vi "Write Scan Log.vi"(8 "error in (no error)":errorcluster, 10 "File Name":string, 11 "Model in":refnum<class "Model.lvclass">) -> (0 "error out":errorcluster, 3 "Model out":refnum<class "Model.lvclass">)   [LabVIEW 2015, in "Model.lvclass"]
uses:
  Model.lvclass
  Typedefs/Write Data File Arguments.ctl
  Typedefs/Write Log Message Arguments.ctl
  Model.lvclass/Model.ctl
  Test Log/Test Log/Test Log.lvclass
  Typedefs/FAMT Typedefs.lvlib
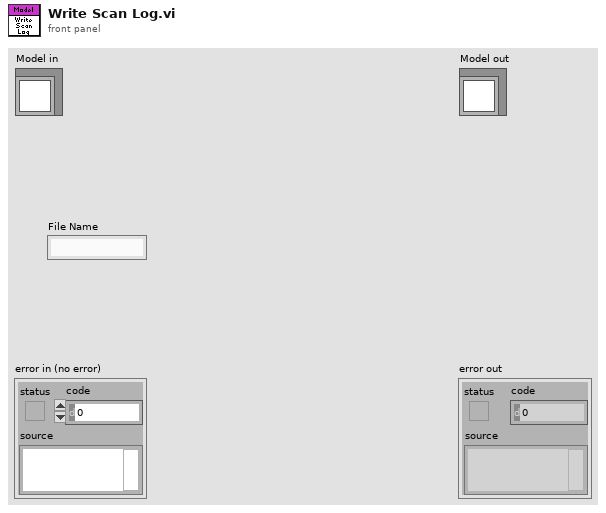
[diagram p1: front panel]
types:
  T1 = typedef "FAMT Typedefs.lvlib/Write Log Message Arguments.ctl" = cluster{"Description":string, "Data File":string}
  T2 = typedef "FAMT Typedefs.lvlib/Write Data File Arguments.ctl" = cluster{"File Name":string, "Output":string[]}
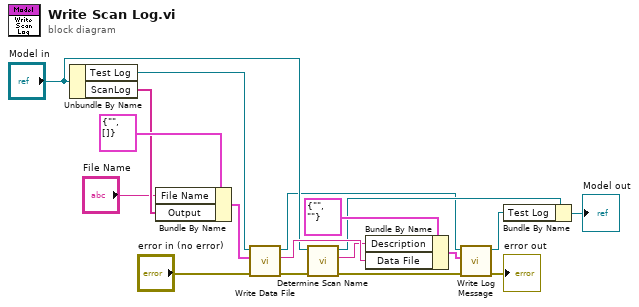
[diagram p0: block diagram]
diagram:
  n1 = Unbundle By Name("Model in") -> ("Test Log"=w18:refnum<class "Test Log.lvclass">, "ScanLog"=w14:string[])
  n2 = Bundle By Name(cluster=T2 {"File Name"="", "Output"=[]} ("WriteDataFileInput"), "File Name"="File Name", "Output"=w14) -> (w15:T2)
  n3 = call-dynamic "Write Data File.vi"("error in (no error)"="error in (no error)", "Write Data File Arguments"=w15, "Test Log in"=w18) -> ("error out"=w3:errorcluster, "Relative Path"=w10:string, "Test Log out"=w6:refnum<class "Test Log.lvclass">)  [unwired: 6 in]
  n4 = call "Determine Scan Name.vi"("error in (no error)"=w3, "Model in"="Model in") -> ("error out"=w2:errorcluster, "Scan Name"=w9:string, "Model out"=w7:refnum<class "Model.lvclass">)  [unwired: 7 in]
  n5 = Bundle By Name(cluster=T1 {"Description"="", "Data File"=""} ("WriteLogMessageInput"), "Description"=w9, "Data File"=w10) -> (w11:T1)
  n6 = call-dynamic "Write Log Message.vi"("error in (no error)"=w2, "Write Log Message Arguments"=w11, "Test Log in"=w6) -> ("error out"=→"error out":errorcluster, "Test Log out"=w5:refnum<class "Test Log.lvclass">)  [unwired: 7 in]
  n7 = Bundle By Name(cluster=w7, "Test Log"=w5) -> (→"Model out":refnum<class "Model.lvclass">)
